vi "U64_Read.vi"(8 "error in (no error)":errorcluster, 9 "Default":u64, 11 "Tag Name":string) -> (0 "error out":errorcluster, 1 "Value":u64)   [LabVIEW 2010, in "Current Value Table.lvlib"]
doc: "This VI will read the data associated with a single tag. This VI will always look up the tag index if the name changes, or if index lookup failed previously (resulting in an error). This combines the functionality of the CVT2 VIs for reads and static reads."
uses:
  Current Value Table.lvlib
  FGVs/Tag Memory Methods.ctl
  Type Defs/Memory Commands.ctl
  U64_Type To Enum.vi
  FGVs/CVT Globals.vi
  U64_Memory Block.vi
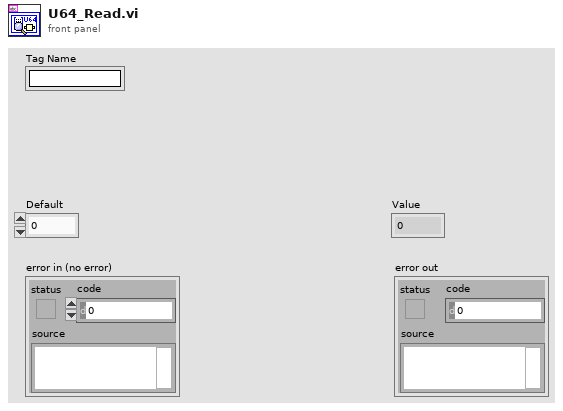
[diagram p1: front panel]
types:
  T1 = typedef "Current Value Table.lvlib/Tag Memory Methods.ctl" = enum16{"Clear", "Read Tag Index", "Read Tag Indices", "Generate Group", "Add Tag", "Overwrite Tag", "Read Description", "Get Stored Tags"}
  T2 = typedef "Current Value Table.lvlib/Data Types.ctl" = enum16{"Double", "Single", "I64", "I32", "I16", "I8", "U64", "U32", "U16", "U8", "String", "Boolean", "Array of U8", "Array of U16", "Array of U32", "Array of U64", "Array of I64", "Array of I32", "Array of I16", "Array of I8", "Array of Double", "Array of Single", "Array of Boolean", "Array of String"}
  T3 = typedef "Current Value Table.lvlib/Memory Commands.ctl" = enum16{"Init", "Add Data", "Read", "Read Group", "Read All", "Write", "Write Group", "Get Size"}
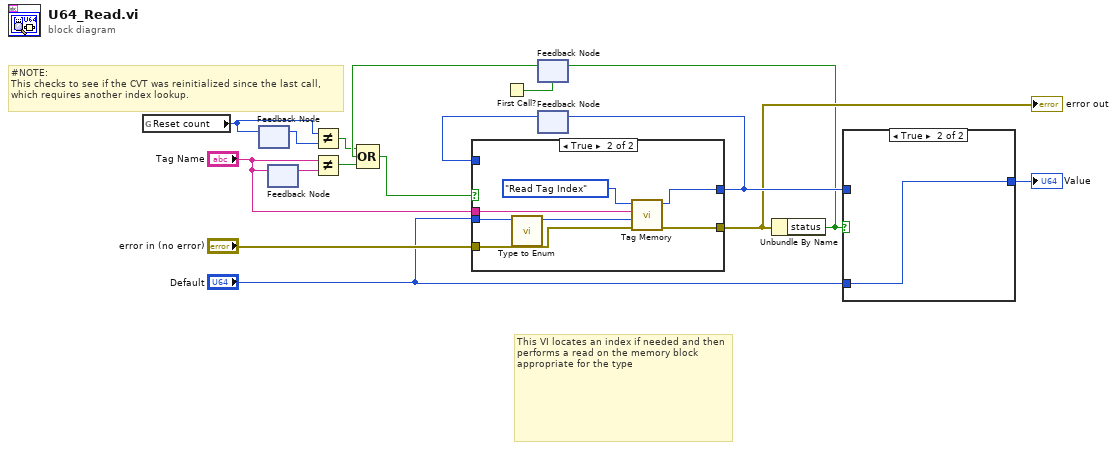
[diagram p0: block diagram]
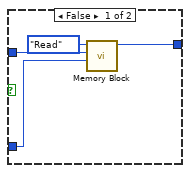
[diagram p2: hidden frame]
diagram:
  # "#NOTE:\nThis checks to see if the CVT was reinitialized since the last call,\nwhich requires another index lookup."
  # "This VI locates an index if needed and then performs a read on the memory block appropriate for the type"
  n1 = global read "CVT Globals.vi" "Reset count"() -> (w2:u32)
  n2 = feedback #1() -> (w3:u32)  [unwired: 1 in]
  n3 = feedback-in #1(w2) -> ()
  n4 = feedback #2() -> (w15:string)  [unwired: 1 in]
  n5 = feedback-in #2("Tag Name") -> ()
  n6 = Not Equal?(x=w2, y=w3) -> (x != y?=w1:bool)
  n7 = Not Equal?(x="Tag Name", y=w15) -> (x != y?=w8:bool)
  n8 = First Call?() -> (First Call?: T/F=w4:bool)
  n9 = feedback #3(w4) -> (w6:bool)
  n10 = Compound Arithmetic op=OR(w1, w6, w8) -> (w5:bool)
  n11 = feedback #4() -> (w14:i32)  [unwired: 1 in]
  n12 = case shown="True" w5 {
    tunnel: [w18 w24] -> w9
    tunnel: "error in (no error)" -> [w18 w19]
    tunnel: [w17 w23] -> w13
    tunnel: w14 -> [w17 _]
    tunnel: "Default" -> [_ w25]
    tunnel: "Tag Name" -> [_ w20]
    frame False {
      # "Reuse Index"
    }
    frame True {
      n13 = call-poly "Type to Enum.vi"("Default"=w25) -> ("Data Type Enum"=w22:T2)  [unwired: 10 in]
      n14 = call "Tag Memory.vi"("error in (no error)"=w19, "Expected Type"=w22, "Tag"=w20, "Method"=Tag_Memory_Methods."Read Tag Index") -> ("error out"=w24:errorcluster, "Index Out"=w23:i32)  [unwired: 2 in, 4 out]
    }
  }
  "error out" <- w9
  n15 = feedback-in #4(w13) -> ()
  n16 = Unbundle By Name(w9) -> ("status"=w7:bool)
  n17 = feedback-in #3(w7) -> ()
  n18 = case shown="True" w7 {
    tunnel: w13 -> [w28 _]
    tunnel: "Default" -> [w27 w30]
    tunnel: [w26 w30] -> w10
    frame False {
      n19 = call-poly "Memory Block.vi"("Value"=w27, "Index"=w28, "Method"=Memory_Commands."Read") -> ("Value Out"=w26:u64)  [unwired: 6 in, 2 out]
    }
    frame True {
    }
  }
  "Value" <- w10
